vi "Reset Meas v 1.vi"   [LabVIEW 2013]
panel:
  # "RESET BUSY"
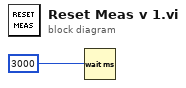
[diagram p0: block diagram]
diagram:
  n1 = Wait (ms)(milliseconds to wait=3000) -> ()  [unwired: 1 out]
